vi "TimingFilestoRegressors.vi"(6 "Uniform Event Offset (s)":dbl, 7 "Array of Basis Functions":dbl[][](array[numeric]), 9 "Array of Timing Files":path[](array[path]), 10 "dt":dbl, 11 "Total Number of Samples":i32) -> (3 "Array of Regressors":dbl[][](array[numeric]))   [LabVIEW 2013]
uses:
  <vilib>/Analysis/2dsp.llb/1D Convolution (DBL).vi
  <vilib>/Utility/file.llb/Read From Spreadsheet File (DBL).vi
  <vilib>/Analysis/NI_AALPro.lvlib
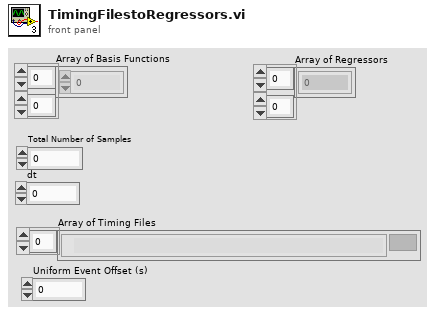
[diagram p1: front panel]
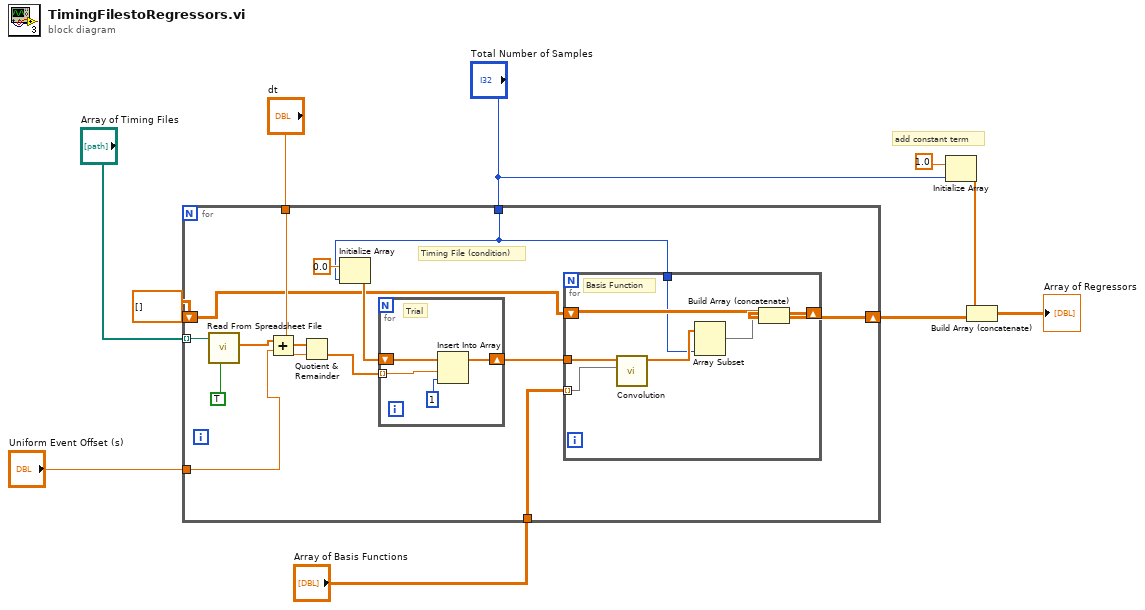
[diagram p0: block diagram]
diagram:
  # "add constant term"
  n1 = for {
    tunnel: "Array of Timing Files" -> [w24] mode=indexing
    shift-right: [w15] -> w2
    shift-left: dbl[][] [] -> [w16]
    tunnel: "Total Number of Samples" -> [w14]
    tunnel: "dt" -> [w22]
    tunnel: "Array of Basis Functions" -> [w18]
    tunnel: "Uniform Event Offset (s)" -> [w11]
    # "Timing File (condition)"
    n2 = call-poly <vilib>:"Read From Spreadsheet File.vi"("transpose (no:F)"=TRUE, "file path (dialog if empty)"=w24) -> ("first row"=w12:dbl[])  [unwired: 5 in, 4 out]
    n3 = Add(x=w12, y=w11) -> (x+y=w13:dbl[])
    n4 = Quotient & Remainder(x=w13, y=w22) -> (floor(x/y)=w19:dbl[])  [unwired: 1 out]
    n5 = Initialize Array(0.0 ("element"), w14) -> (w20:dbl[])
    n6 = for {
      shift-right: [w26] -> w17
      shift-left: w20 -> [w28]
      tunnel: w19 -> [w25] mode=indexing
      # "Trial"
      n7 = Insert Into Array(array=w28, index=w25, new element=1) -> (w26:dbl[])
    }
    n8 = for {
      tunnel: w18 -> [w34] mode=indexing
      tunnel: w17 -> [w35]
      shift-right: [w33] -> w15
      shift-left: w16 -> [w32]
      tunnel: w14 -> [w30]
      # "Basis Function"
      n9 = call-poly <vilib>:"Convolution.vi"("Y"=w34, "X"=w35) -> ("X * Y"=w31:dbl[])  [unwired: 8 in, 1 out]
      n10 = Array Subset(array=w31, length=w30) -> (w29:dbl[])  [unwired: 1 in]
      n11 = Build Array (concatenate)(w32, w29) -> (w33:dbl[][])
    }
  }
  n12 = Initialize Array(1.0 ("element"), "Total Number of Samples") -> (w4:dbl[])
  n13 = Build Array (concatenate)(w4, w2) -> (→"Array of Regressors":dbl[][])
